vi "appendDataFile.vi"(8 "error in (no error)":errorcluster, 10 "read buffer":string, 11 "Byte Stream File in":refnum<file>) -> (0 "error out":errorcluster)   [LabVIEW 2019]
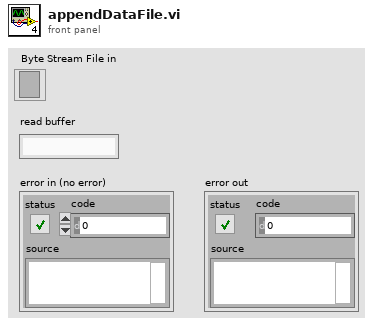
[diagram p1: front panel]
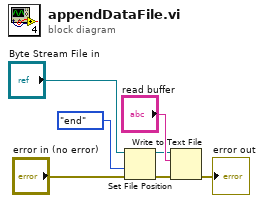
[diagram p0: block diagram]
diagram:
  n1 = Set File Position(refnum="Byte Stream File in", from (0:start)=enum16{"start", "end", "current"}."end", error in="error in (no error)") -> (refnum out=w1:refnum<file>, error out=w3:errorcluster)  [unwired: 1 in]
  n2 = Write to Text File(file (use dialog)=w1, text="read buffer", error in=w3) -> (error out=→"error out":errorcluster)  [unwired: 1 in, 2 out]
